vi "Yokogawa - collect measurements for output.vi"(9 "Normal Measurements":dbl[](array[numeric]), 10 "Waveforms In":waveform(dbl)[](array[waveform]), 11 "Harmonic Measurements":dbl[](array[numeric])) -> (3 "Electrical Data Out":T1={"Time Stamp"=timestamp(0 s since 1904-01-01), "Temperature (C)"=0.0, "Electrical Data"=[["   NaN", "   NaN", "   NaN", "   NaN"], ["   NaN", "   NaN", "   NaN", "   NaN"], ["   NaN", "   NaN", "   NaN", "   NaN"], ["   NaN", "   NaN", "   NaN", "   NaN"], ["   NaN", "   NaN", "   NaN", "   NaN"], ["   NaN", "   NaN", "   NaN", "   NaN"], ["   NaN", "   NaN", "   NaN", "   NaN"], ["   NaN", "   NaN", "   NaN", "   NaN"], ["   NaN", "   NaN", "   NaN", "   NaN"], ["   NaN", "   NaN", "   NaN", "   NaN"]], "Waveform Graph"=[]})   [LabVIEW 2013, in "YKPZ400 Acquisition.lvlib"]
uses:
  controls/electrical2.ctl
  YKPZ400 Acquisition.lvlib
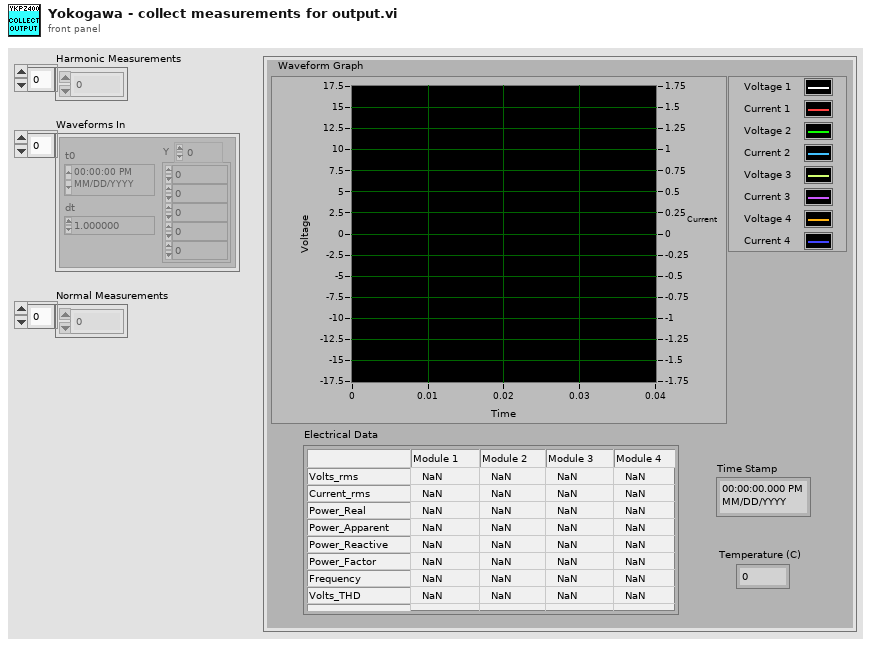
[diagram p1: front panel]
types:
  T1 = typedef "electrical2.ctl" = cluster{"Time Stamp":timestamp, "Temperature (C)":dbl, "Electrical Data":string[][], "Waveform Graph":waveform(dbl)[]}
  T2 = cluster{"seconds since 1Jan1904":timestamp, dbl, string[][], "Waveforms In":waveform(dbl)[]}
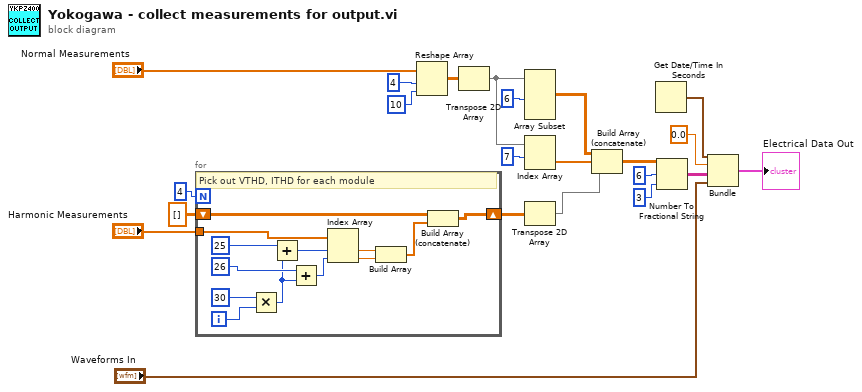
[diagram p0: block diagram]
diagram:
  n1 = for {
    N: 4 -> [_]
    tunnel: "Harmonic Measurements" -> [w26]
    shift-right: [w24] -> w20
    shift-left: dbl[][] [] -> [w23]
    i -> [w35]
    # "Pick out VTHD, ITHD for each module"
    n2 = Multiply(x=30, y=w35) -> (x*y=w31:i32)
    n3 = Add(x=25, y=w31) -> (x+y=w30:i32)
    n4 = Add(x=26, y=w31) -> (x+y=w29:i32)
    n5 = Index Array(array=w26, index #1=w30, index #2=w29) -> (element #1=w28:dbl, element #2=w27:dbl)
    n6 = Build Array(w28, w27) -> (w25:dbl[])
    n7 = Build Array (concatenate)(w23, w25) -> (w24:dbl[][])
  }
  n8 = Reshape Array("Normal Measurements", 4 ("dimension size"), 10 ("dimension size")) -> (w4:dbl[][])
  n9 = Transpose 2D Array(2D array=w4) -> (transposed array=w17:dbl[][])
  n10 = Array Subset(array=w17, length (row)=6 ("length")) -> (w16:dbl[][])  [unwired: 3 in]
  n11 = Index Array(array=w17, index (row)=7) -> (element=w19:dbl[])  [unwired: 1 in]
  n12 = Transpose 2D Array(2D array=w20) -> (transposed array=w21:dbl[][])
  n13 = Build Array (concatenate)(w16, w19, w21) -> (w22:dbl[][])
  n14 = Get Date/Time In Seconds() -> (seconds since 1Jan1904=w7:timestamp)
  n15 = Number To Fractional String(number=w22, width (-)=i16 6, precision (6)=i16 3) -> (F-format string=w9:string[][])  [unwired: 1 in]
  n16 = Bundle("seconds since 1Jan1904"=w7, 0.0, w9, "Waveforms In"="Waveforms In") -> (→"Electrical Data Out":T2)  [unwired: 1 in]
